vi "SetCalculateFormat.vi"(8 "Error In":errorcluster, 10 "Calculate Format Elements":T1[](array[typedef]), 11 "Keithley 6482 In":refnum<visa-resource-name>) -> (0 "Error Out":errorcluster, 3 "Keithley 6482 Out":refnum<visa-resource-name>)   [LabVIEW 8.6, in "Keithley-6482-Visa.lvlib"]
uses:
  Keithley-6482-Visa.lvlib
  Controls/CalculateFormatElement.ctl
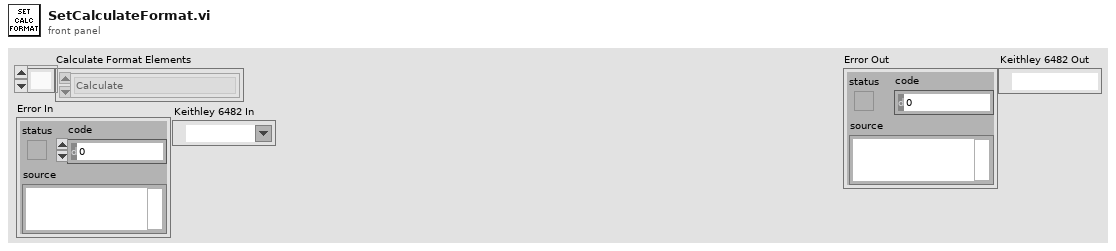
[diagram p1: front panel]
types:
  T1 = typedef "Keithley-6482-Visa.lvlib/CalculateFormatElement.ctl" = enum16{"Calculate", "Time", "Status"}
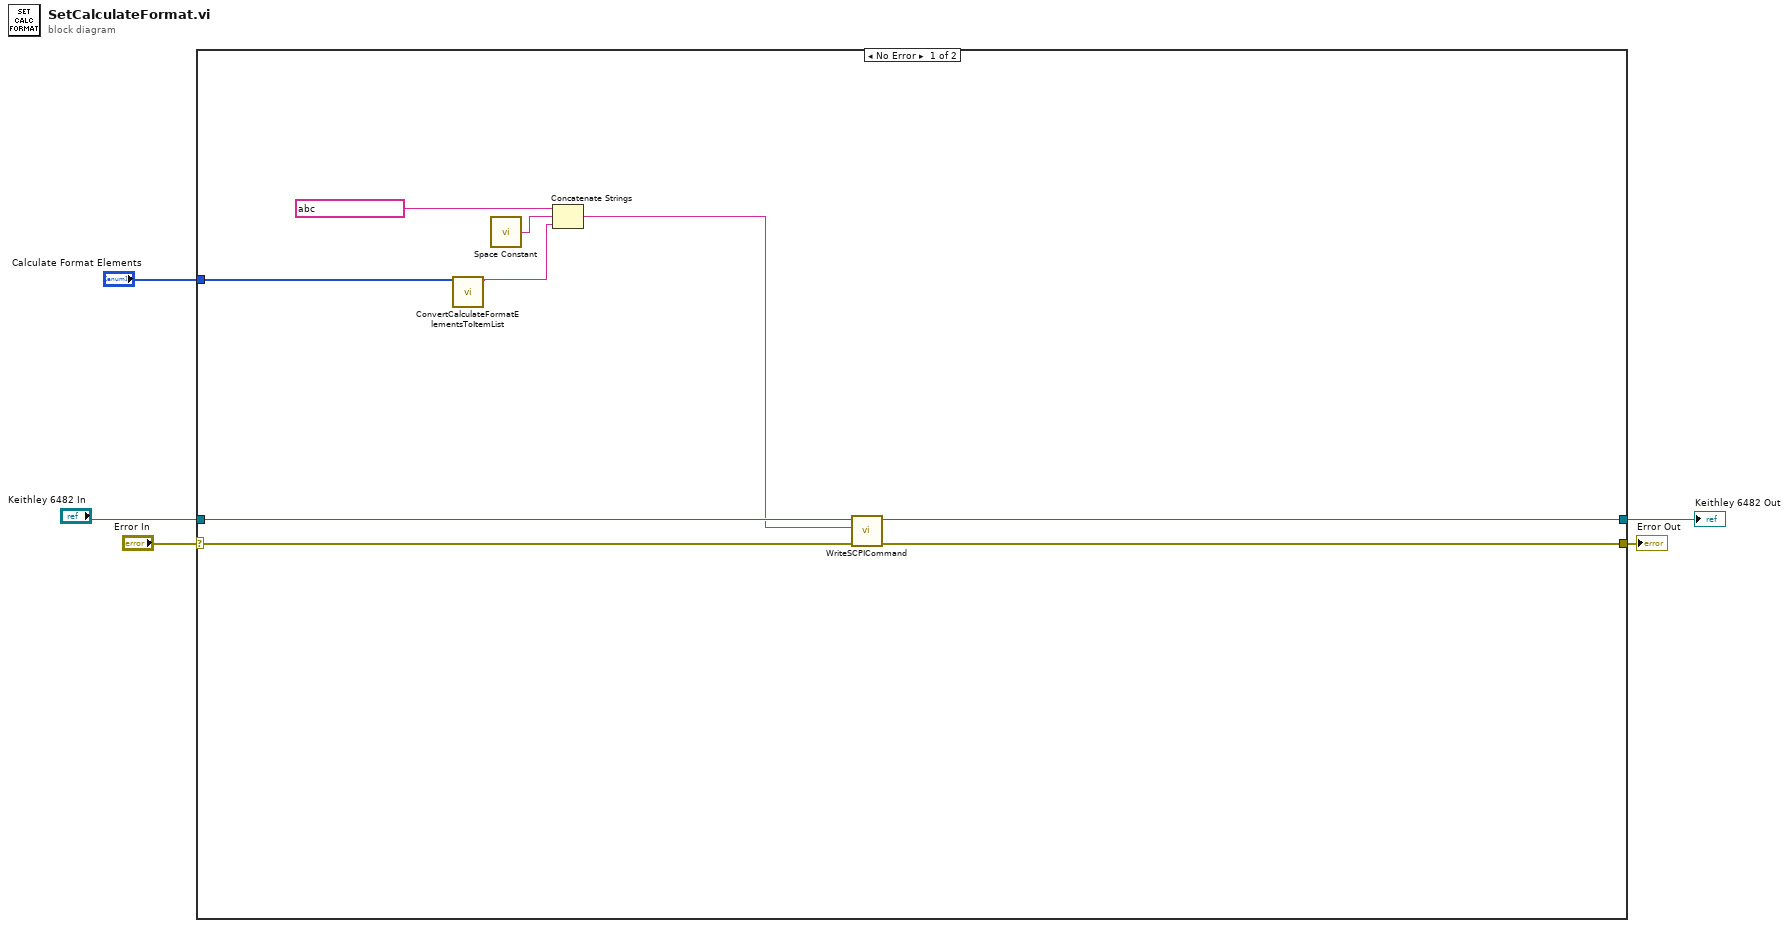
[diagram p0: block diagram]
diagram:
  n1 = case shown="No Error" "Error In" {
    selector: "Error In" -> [w14 w15]
    tunnel: [w13 w15] -> w4
    tunnel: [w12 w16] -> w3
    tunnel: "Keithley 6482 In" -> [w11 w16]
    tunnel: "Calculate Format Elements" -> [w7 _]
    frame #0 {
      n2 = call "ConvertCalculateFormatElementsToItemList.vi"("Calculate Format Elements"=w7) -> ("Item List"=w6:string)  [unwired: 10 in]
      n3 = call <vilib>:"Space Constant.vi"() -> ("String"=w9:string)
      n4 = Concatenate Strings(string ?, w9, w6) -> (w8:string)
      n5 = call "WriteSCPICommand.vi"("Error In"=w14, "SCPI Command"=w8, "Keithley 6482 In"=w11) -> ("Error Out"=w13:errorcluster, "Keithley 6482 Out"=w12:refnum<visa-resource-name>)  [unwired: 7 in]
    }
    frame #1 {
    }
  }
  "Error Out" <- w4
  "Keithley 6482 Out" <- w3
